vi "HoldData_FGV.vi"(7 "HoldData_mods":T1, 8 "error in":errorcluster, 11 "DataIn":variant) -> (0 "error out":errorcluster, 3 "DataOut":variant)   [LabVIEW 2017]
uses:
  HoldData_mods.ctl
  HoldData_data.ctl
  DataForColision.ctl
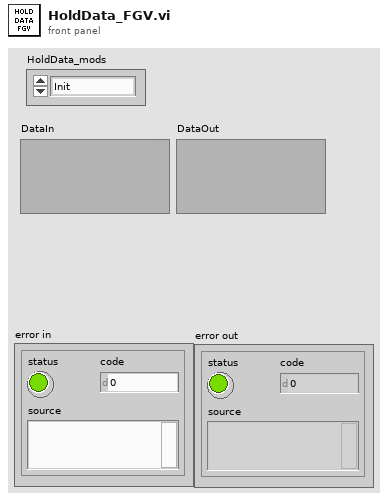
[diagram p1: front panel]
types:
  T1 = typedef "HoldData_mods.ctl" = enum16{"Init", "NewAster", "UpdateAster", "RemoveAster", "GetAsterData", "NewShoot", "UpdateShoot", "RemoveShoot", "GetShootData", "End"}
  T2 = typedef "HoldData_data.ctl" = cluster{"ShootData":T3[], "AsterData":T3[]}
  T3 = typedef "DataForColision.ctl" = cluster{"X":dbl, "Y":dbl, "Size":dbl, "ID":i32}
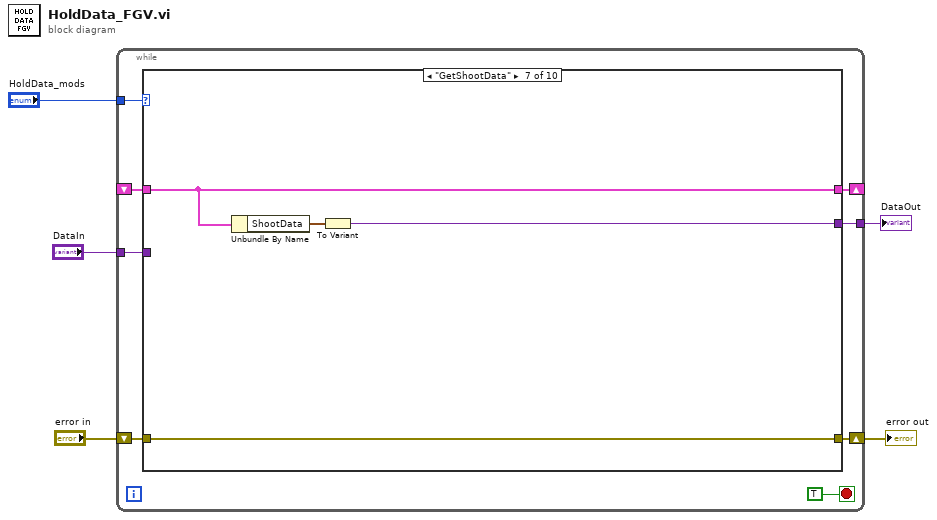
[diagram p0: block diagram]
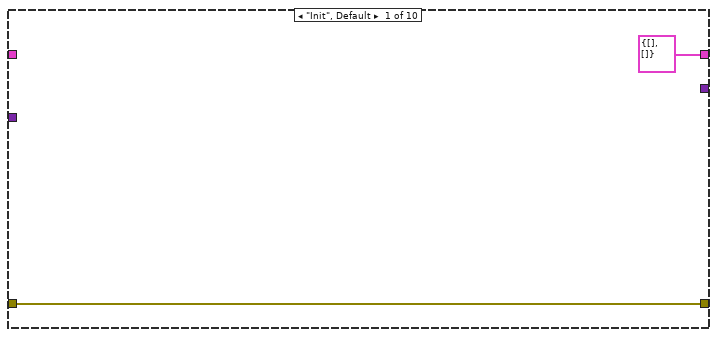
[diagram p2: hidden frame]
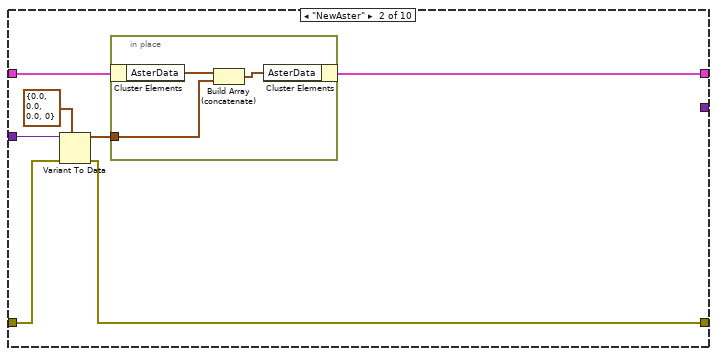
[diagram p3: hidden frame]
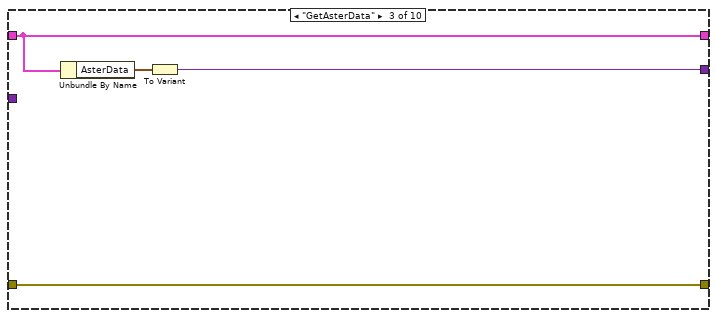
[diagram p4: hidden frame]
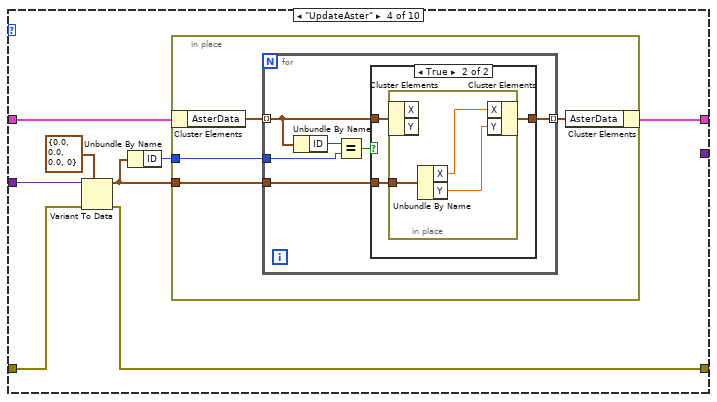
[diagram p5: hidden frame]
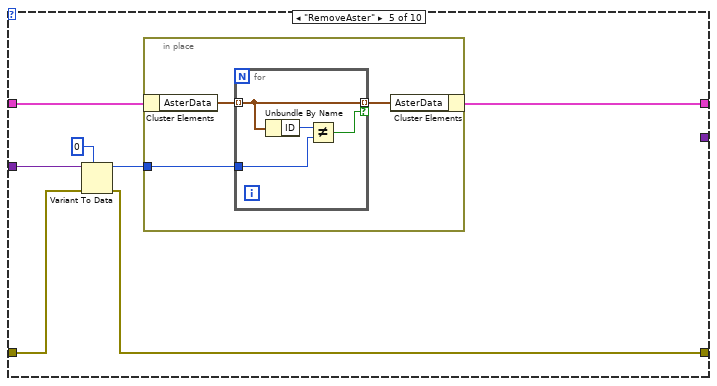
[diagram p7: hidden frame]
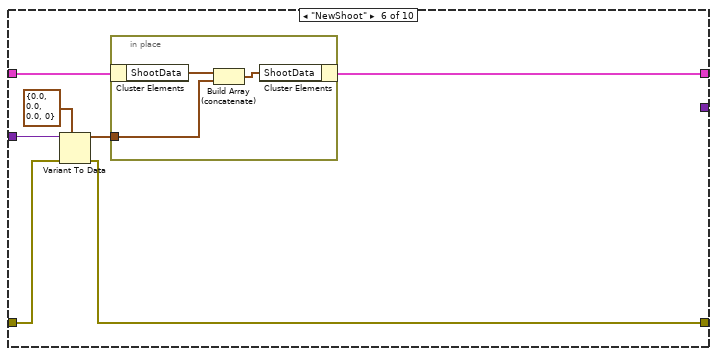
[diagram p8: hidden frame]
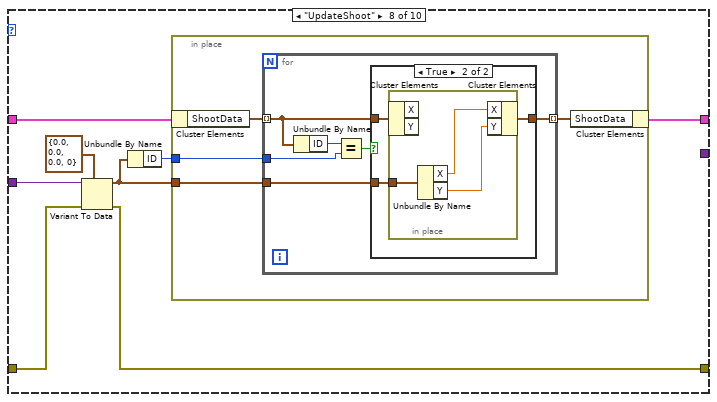
[diagram p9: hidden frame]
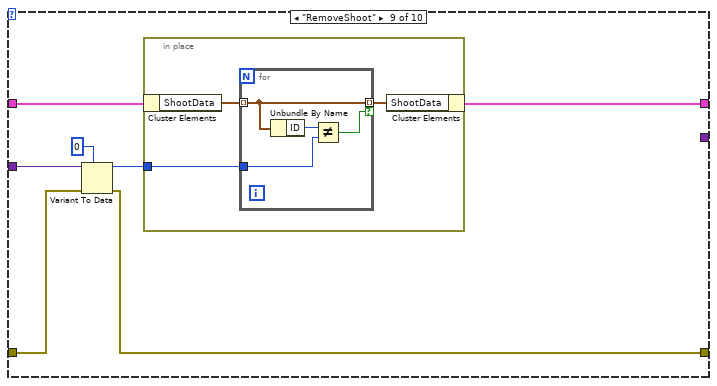
[diagram p11: hidden frame]
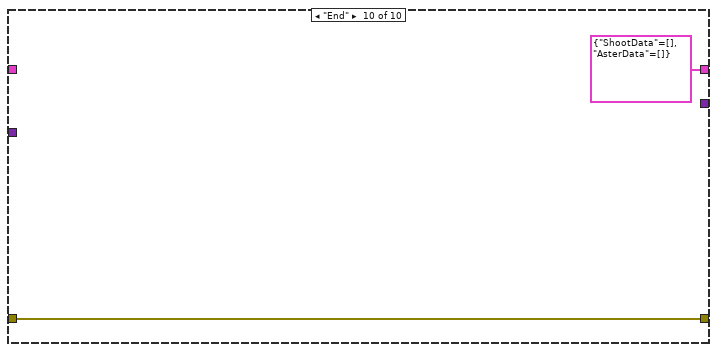
[diagram p12: hidden frame]
diagram:
  n1 = while {
    shift-right: [w9] -> w4
    shift-left: "error in" -> [w13]
    tunnel: "DataIn" -> [w11]
    tunnel: "HoldData_mods" -> [w10]
    shift-right: [w8] -> _
    shift-left: _ -> [w7]
    tunnel: [w6] -> w1
    stop <- TRUE stop-if-true
    n2 = case shown="\"GetShootData\"" w10 {
      tunnel: w13 -> [w15 w21 w26 w35 w60 w74 w79 w88 w113 w123]
      tunnel: w11 -> [_ w22 _ w36 w61 w75 _ w89 w114 _]
      tunnel: [w15 w17 w26 w33 w58 w70 w79 w86 w111 w123] -> w9
      tunnel: [T2 {"ShootData"=[], "AsterData"=[]} ("HoldData_data") w16 w29 w31 w57 w69 w81 w84 w110 T2 {"ShootData"=[], "AsterData"=[]} ("HoldData_data")] -> w8
      tunnel: w7 -> [_ w19 w29 w34 w59 w72 w81 w87 w112 _]
      tunnel: [_ _ w27 _ _ _ w80 _ _ _] -> w6
      frame "Init", Default {
      }
      frame "NewAster" {
        n3 = Variant To Data(error in=w21, type=T3 {"X"=0.0, "Y"=0.0, "Size"=0.0, "ID"=0} ("DataForColision"), Variant=w22) -> (data=w18:T3, error out=w17:errorcluster)
        n4 = in-place {
          in-place-border: w18 -> [w24]
          n5 = in-place-cluster #1(w19) -> ("AsterData"=w25:T3[])
          n6 = Build Array (concatenate)(w25, w24) -> (w23:T3[])
          n7 = in-place-cluster #1("AsterData"=w23) -> (w16:T2)
        }
      }
      frame "GetAsterData" {
        n8 = Unbundle By Name(w29) -> ("AsterData"=w28:T3[])
        n9 = To Variant(anything=w28) -> (Variant=w27:variant)
      }
      frame "UpdateAster" {
        n10 = Variant To Data(error in=w35, type=T3 {"X"=0.0, "Y"=0.0, "Size"=0.0, "ID"=0} ("DataForColision"), Variant=w36) -> (data=w30:T3, error out=w33:errorcluster)
        n11 = Unbundle By Name(w30) -> ("ID"=w32:i32)
        n12 = in-place {
          in-place-border: w32 -> [w40]
          in-place-border: w30 -> [w38]
          n13 = in-place-cluster #2(w34) -> ("AsterData"=w41:T3[])
          n14 = for {
            tunnel: w41 -> [w47] mode=indexing
            tunnel: w40 -> [w45]
            tunnel: [w44] -> w39 mode=indexing
            tunnel: w38 -> [w42]
            n15 = Unbundle By Name(w47) -> ("ID"=w46:i32)
            n16 = Equal?(x=w46, y=w45) -> (x = y?=w43:bool)
            n17 = case shown="True" w43 {
              tunnel: w47 -> [w48 w51]
              tunnel: [w48 w50] -> w44
              tunnel: w42 -> [_ w49]
              frame False {
              }
              frame True {
                n18 = in-place {
                  in-place-border: w49 -> [w54]
                  n19 = in-place-cluster #3(w51) -> ()  [unwired: 2 out]
                  n20 = Unbundle By Name(w54) -> ("X"=w53:dbl, "Y"=w52:dbl)
                  n21 = in-place-cluster #3("X"=w53, "Y"=w52) -> (w50:T3)
                }
              }
            }
          }
          n22 = in-place-cluster #2("AsterData"=w39) -> (w31:T2)
        }
      }
      frame "RemoveAster" {
        n23 = Variant To Data(error in=w60, type=0, Variant=w61) -> (data=w55:i32, error out=w58:errorcluster)
        n24 = in-place {
          in-place-border: w55 -> [w63]
          n25 = in-place-cluster #4(w59) -> ("AsterData"=w64:T3[])
          n26 = for {
            tunnel: w64 -> [w65] mode=indexing
            tunnel: w63 -> [w67]
            tunnel: [w65] -> w62 mode=indexing if=w66
            n27 = Unbundle By Name(w65) -> ("ID"=w68:i32)
            n28 = Not Equal?(x=w68, y=w67) -> (x != y?=w66:bool)
          }
          n29 = in-place-cluster #4("AsterData"=w62) -> (w57:T2)
        }
      }
      frame "NewShoot" {
        n30 = Variant To Data(error in=w74, type=T3 {"X"=0.0, "Y"=0.0, "Size"=0.0, "ID"=0} ("DataForColision"), Variant=w75) -> (data=w71:T3, error out=w70:errorcluster)
        n31 = in-place {
          in-place-border: w71 -> [w77]
          n32 = in-place-cluster #5(w72) -> ("ShootData"=w78:T3[])
          n33 = Build Array (concatenate)(w78, w77) -> (w76:T3[])
          n34 = in-place-cluster #5("ShootData"=w76) -> (w69:T2)
        }
      }
      frame "GetShootData" {
        n35 = Unbundle By Name(w81) -> ("ShootData"=w82:T3[])
        n36 = To Variant(anything=w82) -> (Variant=w80:variant)
      }
      frame "UpdateShoot" {
        n37 = Variant To Data(error in=w88, type=T3 {"X"=0.0, "Y"=0.0, "Size"=0.0, "ID"=0} ("DataForColision"), Variant=w89) -> (data=w83:T3, error out=w86:errorcluster)
        n38 = Unbundle By Name(w83) -> ("ID"=w85:i32)
        n39 = in-place {
          in-place-border: w85 -> [w93]
          in-place-border: w83 -> [w91]
          n40 = in-place-cluster #6(w87) -> ("ShootData"=w94:T3[])
          n41 = for {
            tunnel: w94 -> [w100] mode=indexing
            tunnel: w93 -> [w98]
            tunnel: [w97] -> w92 mode=indexing
            tunnel: w91 -> [w95]
            n42 = Unbundle By Name(w100) -> ("ID"=w99:i32)
            n43 = Equal?(x=w99, y=w98) -> (x = y?=w96:bool)
            n44 = case shown="True" w96 {
              tunnel: w100 -> [w101 w104]
              tunnel: [w101 w103] -> w97
              tunnel: w95 -> [_ w102]
              frame False {
              }
              frame True {
                n45 = in-place {
                  in-place-border: w102 -> [w107]
                  n46 = in-place-cluster #7(w104) -> ()  [unwired: 2 out]
                  n47 = Unbundle By Name(w107) -> ("X"=w106:dbl, "Y"=w105:dbl)
                  n48 = in-place-cluster #7("X"=w106, "Y"=w105) -> (w103:T3)
                }
              }
            }
          }
          n49 = in-place-cluster #6("ShootData"=w92) -> (w84:T2)
        }
      }
      frame "RemoveShoot" {
        n50 = Variant To Data(error in=w113, type=0, Variant=w114) -> (data=w108:i32, error out=w111:errorcluster)
        n51 = in-place {
          in-place-border: w108 -> [w116]
          n52 = in-place-cluster #8(w112) -> ("ShootData"=w117:T3[])
          n53 = for {
            tunnel: w117 -> [w118] mode=indexing
            tunnel: w116 -> [w120]
            tunnel: [w118] -> w115 mode=indexing if=w119
            n54 = Unbundle By Name(w118) -> ("ID"=w121:i32)
            n55 = Not Equal?(x=w121, y=w120) -> (x != y?=w119:bool)
          }
          n56 = in-place-cluster #8("ShootData"=w115) -> (w110:T2)
        }
      }
      frame "End" {
      }
    }
  }
  "error out" <- w4
  "DataOut" <- w1
